vi "Create Events Refs.vi"(11 "Hello World Event in":refnum<class "Hello World Event.lvclass">) -> (3 "Hello World Event out":refnum<class "Hello World Event.lvclass">)   [LabVIEW 2021, in "Hello World Event.lvlib" / "Hello World Event.lvclass"]
uses:
  Hello World Event.lvclass
  Hello World Event.lvclass/Hello World Event.ctl
  C:/git/jettl/src/Actor/Actor/Actor.lvclass
  C:/git/jettl/src/Actor/Msgs/Setup/Setup/Setup.lvclass
  C:/git/jettl/src/Actor/Msgs/Teardown/Teardown/Teardown.lvclass
  C:/git/jettl/src/Actor/Event Actor/Event Actor.lvclass
  C:/git/jettl/src/Actor/Msgs/Update Queue Nested/Update Queue Nested/Update Queue Nested.lvclass
  C:/git/jettl/src/Hello World/Hello World Event/Hello World Event/Hello World Event.lvclass
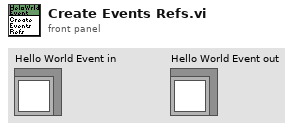
[diagram p1: front panel]
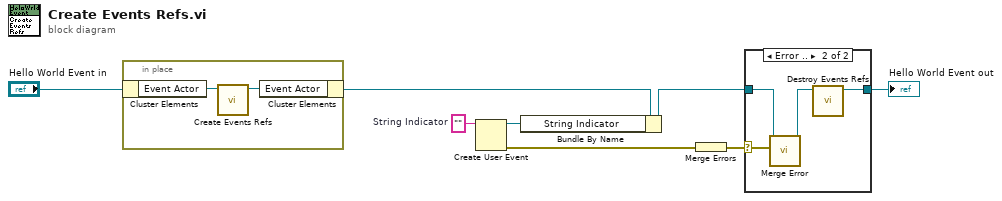
[diagram p0: block diagram]
diagram:
  w7 = ""  # String Indicator
  n1 = in-place {
    n2 = in-place-cluster #1("Hello World Event in") -> ("Event Actor"=w10:refnum<class "Event Actor.lvclass">)
    n3 = call-dynamic "Create Events Refs.vi"("Hello World Event in"=w10) -> ("Hello World Event out"=w9:refnum<class "Hello World Event.lvclass">)  [unwired: 10 in]
    n4 = in-place-cluster #1("Event Actor"=w9) -> (w1:refnum<class "Hello World Event.lvclass">)
  }
  n5 = Create User Event(user event datatype=w7) -> (user event=w8:refnum<user-event>, error out=w6:errorcluster)  [unwired: 1 in]
  n6 = Bundle By Name(cluster=w1, "String Indicator"=w8) -> (w4:refnum<class "Hello World Event.lvclass">)
  n7 = Merge Errors(w6) -> (w5:errorcluster)
  n8 = case shown="Error .." w5 {
    selector: w5 -> [_ w15]
    tunnel: [w11 w12] -> w3
    tunnel: w4 -> [w11 w14]
    frame No Error {
    }
    frame Error {
      n9 = call-dynamic "Merge Error.vi"("Error"=w15, "Set Error in"=w14) -> ("Set Error out"=w13:refnum<class "Hello World Event.lvclass">)  [unwired: 9 in]
      n10 = call-dynamic "Destroy Events Refs.vi"("Hello World Event in"=w13) -> ("Hello World Event out"=w12:refnum<class "Hello World Event.lvclass">)  [unwired: 10 in]
    }
  }
  "Hello World Event out" <- w3
